vi "Open Butterfly Spark MAX.vi"(8 "error in (no error)":errorcluster, 9 "Cluster":T6, 10 "Seconds from neutral to full (0)":sgl=0.1, 11 "Idle Mode":T7) -> (0 "error out":errorcluster, 1 "butterfly drive":T1, 2 "right drive":T1, 3 "left drive":T1)   [LabVIEW 2018]
uses:
  <vilib>/Rock Robotics/WPI/MotorControl/WPI_MotorControlDeviceRef.ctl
  <vilib>/Rock Robotics/WPI/MotorControl/WPI_MotorControlType.ctl
  <vilib>/Rock Robotics/SystemInterfaces/DIO/FPGA_DIOPWMChannel.ctl
  <vilib>/Rock Robotics/WPI/PWM/WPI_PWMDeadband.ctl
  <vilib>/Rock Robotics/SystemInterfaces/DIO/FPGA_DIOChannel.ctl
  <vilib>/Rock Robotics/WPI/ThirdParty/REV Robotics/SPARK MAX/Typedef/Spark MAX Idle Mode.ctl
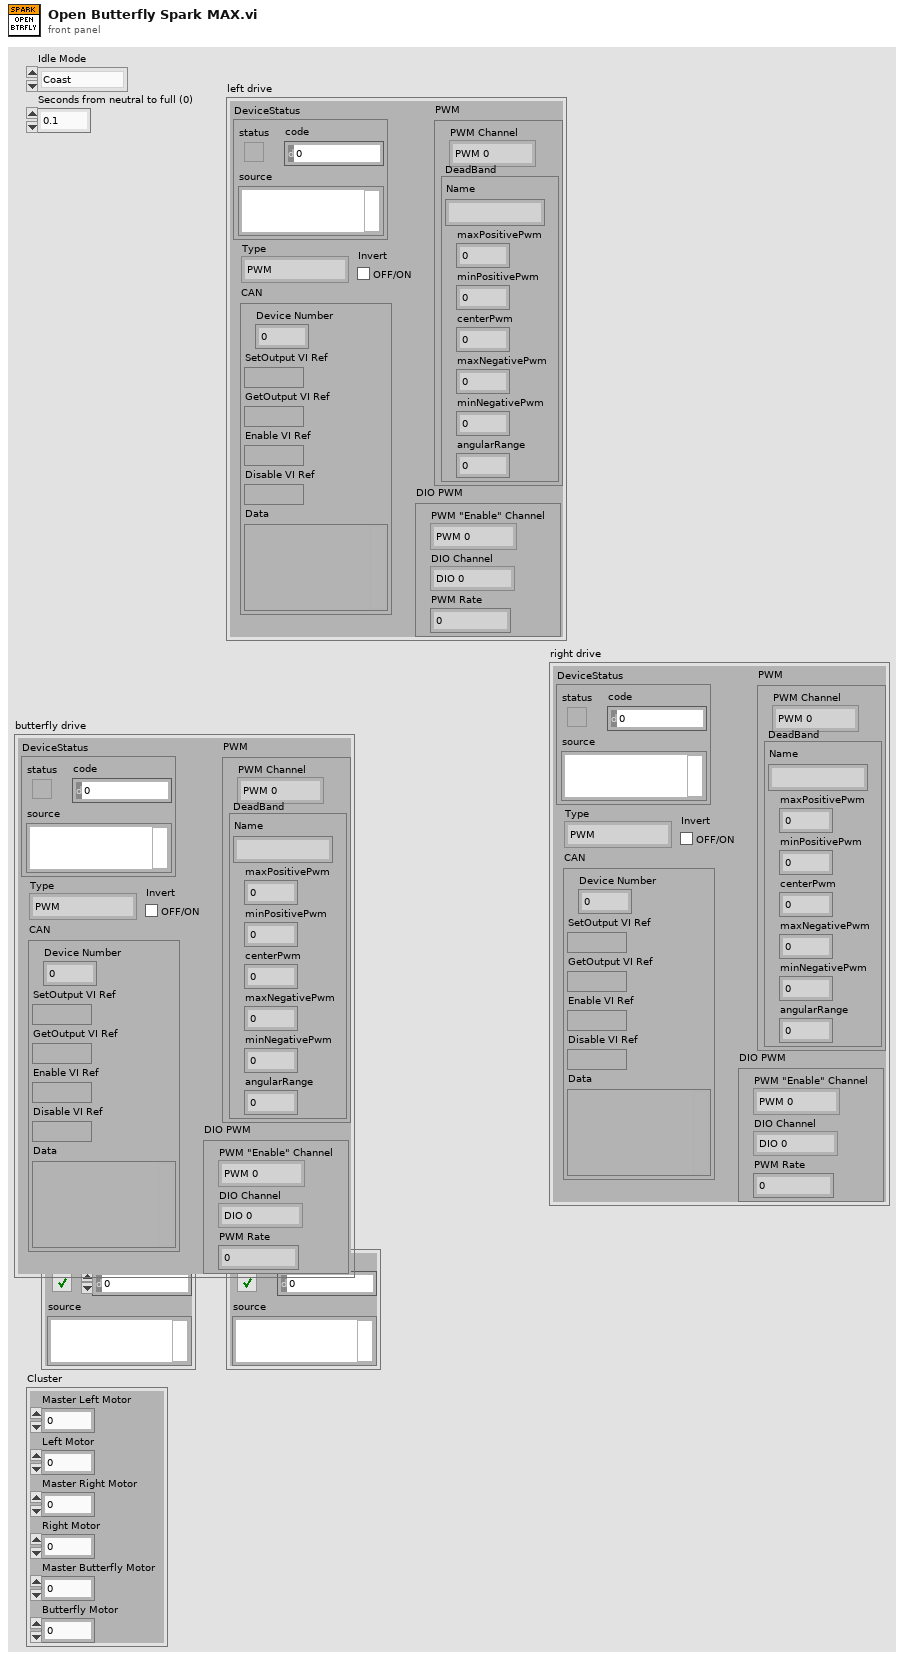
[diagram p1: front panel]
types:
  T1 = typedef "WPI_MotorControlDeviceRef.ctl" = cluster{"DeviceStatus":errorcluster, "Type":T2, "PWM":cluster{"PWM Channel":T3, "DeadBand":T4}, "CAN":cluster{"Device Number":u8, "SetOutput VI Ref":variant, "GetOutput VI Ref":variant, "Enable VI Ref":variant, "Disable VI Ref":variant, "Data":variant}, "Invert":bool, "DIO PWM":cluster{"PWM \"Enable\" Channel":T3, "DIOChannel":T5, "PWM Rate":dbl}}
  T2 = typedef "WPI_MotorControlType.ctl" = enum16{"PWM", "CAN", "DIO PWM"}
  T3 = typedef "FPGA_DIOPWMChannel.ctl" = enum8{"PWM 0", "PWM 1", "PWM 2", "PWM 3", "PWM 4", "PWM 5", "PWM 6", "PWM 7", "PWM 8", "PWM 9", "PWM MXP 0", "PWM MXP 1", "PWM MXP 2", "PWM MXP 3", "PWM MXP 4", "PWM MXP 5", "PWM MXP 6", "PWM MXP 7", "PWM MXP 8", "PWM MXP 9", "Invalid"}
  T4 = typedef "WPI_PWMDeadband.ctl" = cluster{"Name":string, "maxPositivePwm":i32, "minPositivePwm":i32, "centerPwm":i32, "maxNegativePwm":i32, "minNegativePwm":i32, "angularRange":u16}
  T5 = typedef "FPGA_DIOChannel.ctl" = enum8{"DIO 0", "DIO 1", "DIO 2", "DIO 3", "DIO 4", "DIO 5", "DIO 6", "DIO 7", "DIO 8", "DIO 9", "DIO MXP 0", "DIO MXP 1", "DIO MXP 2", "DIO MXP 3", "DIO MXP 4", "DIO MXP 5", "DIO MXP 6", "DIO MXP 7", "DIO MXP 8", "DIO MXP 9", "DIO MXP 10", "DIO MXP 11", "DIO MXP 12", "DIO MXP 13", "DIO MXP 14", "DIO MXP 15", "SPI Port CS1", "SPI Port CS2", "SPI Port CS3", "SPI Port MISO", "SPI Port MOSI", "Invalid"}
  T6 = cluster{"Master Left Motor":u8, "Left Motor":u8, "Master Right Motor":u8, "Right Motor":u8, "Master Butterfly Motor":i32, "Butterfly Motor":i32}
  T7 = typedef "Spark MAX Idle Mode.ctl" = enum16{"Coast", "Brake"}
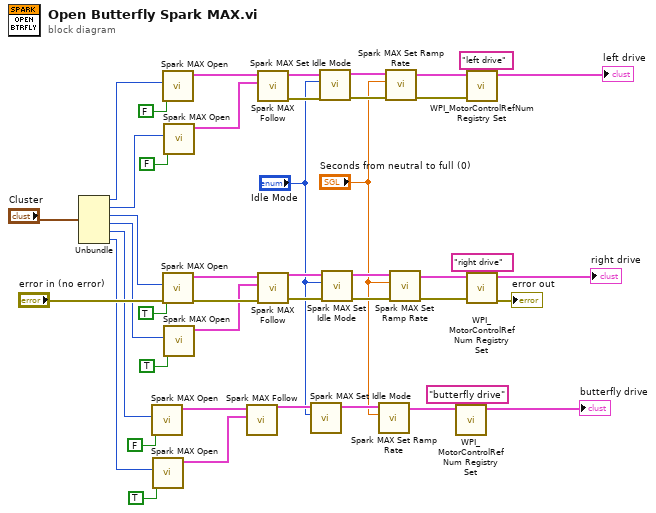
[diagram p0: block diagram]
diagram:
  n1 = Unbundle("Cluster") -> ("Master Left Motor"=w17:u8, "Left Motor"=w16:u8, "Master Right Motor"=w15:u8, "Right Motor"=w14:u8, "Master Butterfly Motor"=w4:i32, "Butterfly Motor"=w3:i32)
  n2 = call <vilib>:"Spark MAX Open.vi"("Invert"=FALSE, "Device Number"=w4) -> ("MotorControlDeviceRef"=w13:T1)  [unwired: 8 in, 1 out]
  n3 = call <vilib>:"Spark MAX Open.vi"("Invert"=TRUE, "Device Number"=w3) -> ("MotorControlDeviceRef"=w9:T1)  [unwired: 8 in, 1 out]
  n4 = call <vilib>:"Spark MAX Open.vi"("Invert"=FALSE, "Device Number"=w17) -> ("MotorControlDeviceRef"=w24:T1)  [unwired: 8 in, 1 out]
  n5 = call <vilib>:"Spark MAX Open.vi"("error in (no error)"="error in (no error)", "Invert"=TRUE, "Device Number"=w15) -> ("error out"=w32:errorcluster, "MotorControlDeviceRef"=w25:T1)  [unwired: 7 in]
  n6 = call <vilib>:"Spark MAX Open.vi"("Invert"=FALSE, "Device Number"=w16) -> ("MotorControlDeviceRef"=w19:T1)  [unwired: 8 in, 1 out]
  n7 = call <vilib>:"Spark MAX Open.vi"("Invert"=TRUE, "Device Number"=w14) -> ("MotorControlDeviceRef"=w29:T1)  [unwired: 8 in, 1 out]
  n8 = call <vilib>:"Spark MAX Follow.vi"("Master Controller"=w9, "MotorControlDeviceRef"=w13) -> ("MotorControlDeviceRef"=w7:T1)  [unwired: 8 in, 1 out]
  n9 = call <vilib>:"Spark MAX Follow.vi"("Master Controller"=w19, "MotorControlDeviceRef"=w24) -> ("error out"=w35:errorcluster, "MotorControlDeviceRef"=w34:T1)  [unwired: 8 in]
  n10 = call <vilib>:"Spark MAX Follow.vi"("error in (no error)"=w32, "Master Controller"=w29, "MotorControlDeviceRef"=w25) -> ("error out"=w37:errorcluster, "MotorControlDeviceRef"=w36:T1)  [unwired: 7 in]
  n11 = call <vilib>:"Spark MAX Set Idle Mode.vi"("Idle Mode"="Idle Mode", "MotorControlDeviceRef in"=w7) -> ("MotorControlDeviceRef out"=w6:T1)  [unwired: 8 in, 1 out]
  n12 = call <vilib>:"Spark MAX Set Idle Mode.vi"("error in (no error)"=w35, "Idle Mode"="Idle Mode", "MotorControlDeviceRef in"=w34) -> ("error out"=w42:errorcluster, "MotorControlDeviceRef out"=w43:T1)  [unwired: 7 in]
  n13 = call <vilib>:"Spark MAX Set Idle Mode.vi"("error in (no error)"=w37, "Idle Mode"="Idle Mode", "MotorControlDeviceRef in"=w36) -> ("error out"=w39:errorcluster, "MotorControlDeviceRef out"=w38:T1)  [unwired: 7 in]
  n14 = call <vilib>:"Spark MAX Set Ramp Rate.vi"("Seconds from neutral to full (0)"="Seconds from neutral to full (0)", "MotorControlDeviceRef in"=w6) -> ("MotorControlDeviceRef"=w5:T1)  [unwired: 8 in, 1 out]
  n15 = call <vilib>:"Spark MAX Set Ramp Rate.vi"("error in (no error)"=w42, "Seconds from neutral to full (0)"="Seconds from neutral to full (0)", "MotorControlDeviceRef in"=w43) -> ("error out"=w44:errorcluster, "MotorControlDeviceRef"=w45:T1)  [unwired: 7 in]
  n16 = call <vilib>:"Spark MAX Set Ramp Rate.vi"("error in (no error)"=w39, "Seconds from neutral to full (0)"="Seconds from neutral to full (0)", "MotorControlDeviceRef in"=w38) -> ("error out"=w40:errorcluster, "MotorControlDeviceRef"=w41:T1)  [unwired: 7 in]
  n17 = call <vilib>:"WPI_MotorControlRefNum Registry Set.vi"("refnum name"="butterfly drive", "MotorControlDevRef"=w5) -> ("MotorControlDevRef"=→"butterfly drive":T1)  [unwired: 8 in, 1 out]
  n18 = call <vilib>:"WPI_MotorControlRefNum Registry Set.vi"("error in (no error)"=w44, "refnum name"="left drive", "MotorControlDevRef"=w45) -> ("MotorControlDevRef"=→"left drive":T1)  [unwired: 7 in, 1 out]
  n19 = call <vilib>:"WPI_MotorControlRefNum Registry Set.vi"("error in (no error)"=w40, "refnum name"="right drive", "MotorControlDevRef"=w41) -> ("error out"=→"error out":errorcluster, "MotorControlDevRef"=→"right drive":T1)  [unwired: 7 in]
